vi "post_dust_event_small.vi"(8 "error in (no error)":errorcluster, 11 "Cluster":T1 {"File Location" items=["Currently Writing"=-3, "Labview Files"=-2, "Mars Data Processing Factility"=-1, "Local Cache "=0, "Old Storage"=1, "Storage"=2]; "Estimate Source" items=["Any Source."=-2, "No Shot"=-1, "Basic Labview Estimate"=0, "IDL Estimate From Andrew"=1, "IDL Estimate From Tobin"=2, "Old Metadata"=3]}) -> (0 "error out":errorcluster, 1 "Experiment Settings":i32, 2 "Dust Event ID":i32, 3 "Test Server":bool)   [LabVIEW 2013]
uses:
  Post_Dust_Event_small.ctl
  Private/Estimate_source.ctl
  Private/File_location.ctl
  <vilib>/addons/database/Auxilliary.llb/DB Tools Cursor Type.ctl
  <vilib>/addons/database/Connection.llb/Conn Execute.vi
  <vilib>/addons/database/Recordset.llb/Rec Fetch Recordset Data (R).vi
  <vilib>/addons/database/Recordset.llb/Rec Destroy - Connection.vi
  <vilib>/addons/database/_DB Variant To Data/Database Variant To Data.xnode
  <vilib>/addons/database/NI_Database_API.lvlib
panel:
  # "Dust Event Small"
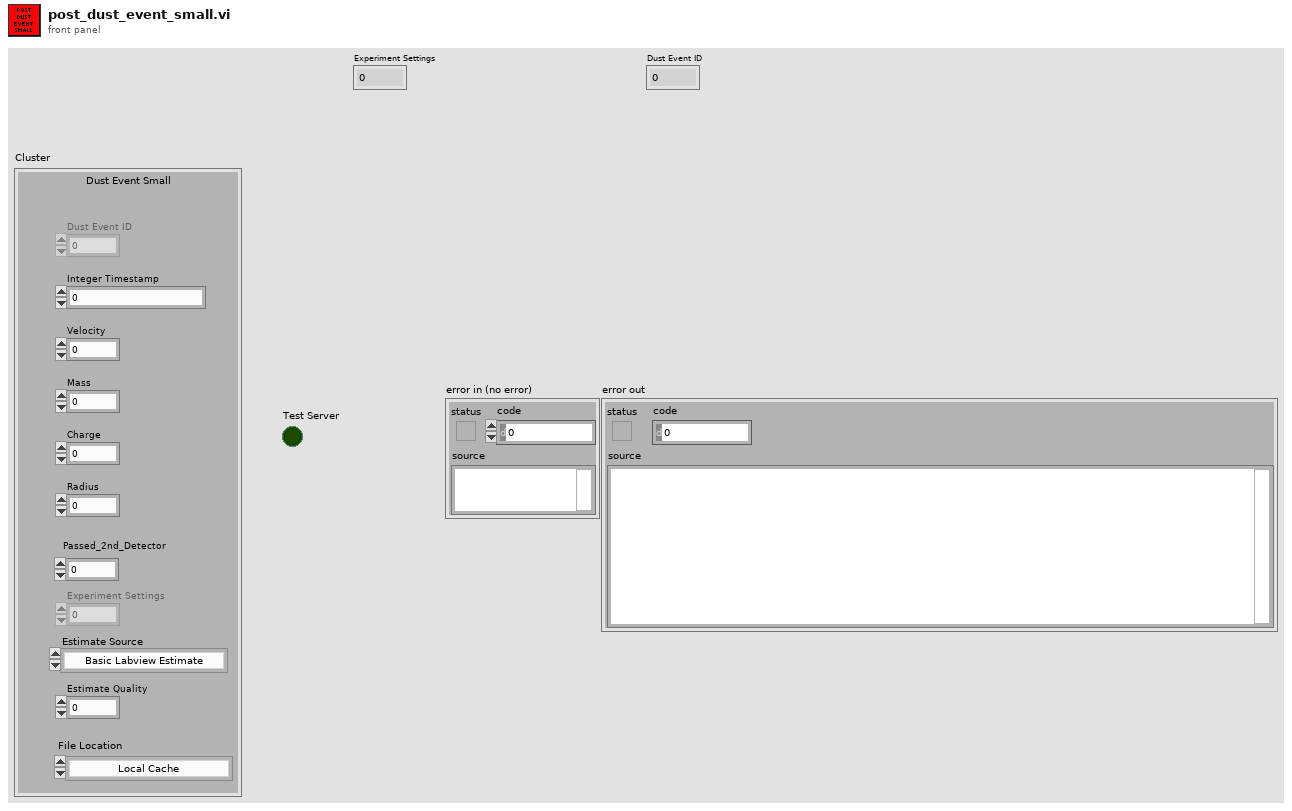
[diagram p1: front panel]
types:
  T1 = typedef "Post_Dust_Event_small.ctl" = cluster{"Dust Event ID":i64, "Integer Timestamp":i64, "Velocity":sgl, "Mass":sgl, "Charge":sgl, "Radius":sgl, "Passed_2nd_Detector":i8, "Experiment Settings":dbl, "Estimate Source":T2, "Estimate Quality":sgl, "File Location":T3, "id_dust_info":dbl}
  T2 = typedef "Estimate_source.ctl" = i8
  T3 = typedef "File_location.ctl" = i8
  T4 = typedef "NI_Database_API.lvlib/DB Tools Cursor Type.ctl" = enum16{"forward-only", "keyset", "dynamic", "static"}
  T5 = typedef "NI_Database_API.lvlib/Conn ObjectReference.ctl" = refnum<k1>
  T6 = typedef "NI_Database_API.lvlib/Rec ObjectReference.ctl" = refnum<k1>
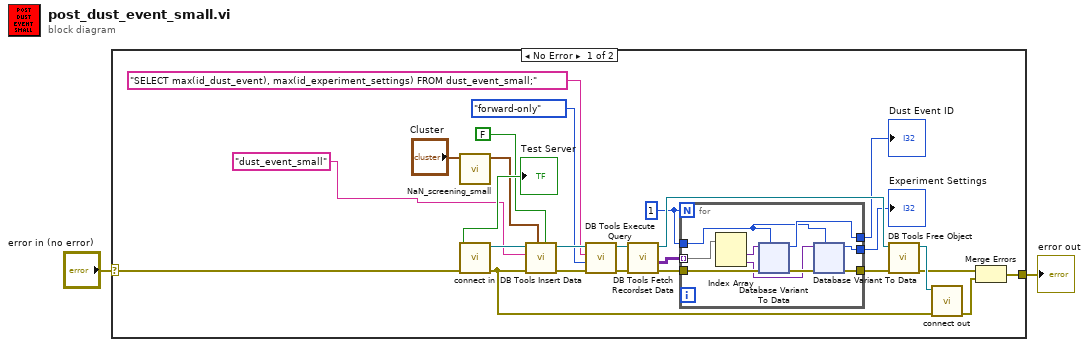
[diagram p0: block diagram]
diagram:
  n1 = case shown="No Error" "error in (no error)" {
    selector: "error in (no error)" -> [w24 w101]
    tunnel: [w21 w101] -> w1
    frame No Error {
      w11 = 1
      n2 = call "NaN_screening_small.vi"("Input"="Cluster") -> ("Output"=w6:T1)  [unwired: 10 in]
      n3 = call "connect in.vi"("error in (no error)"=w24) -> ("error out"=w23:errorcluster, "Database Connection"=w27:T5, "Test Server"=→"Test Server":bool)  [unwired: 6 in]
      n4 = call <vilib>:"DB Tools Insert Data.vi"("create table? (F)"=FALSE, "data"=w6, "error in (no error)"=w23, "table"="dust_event_small", "connection reference"=w27) -> ("error out"=w5:errorcluster, "connection reference out"=w18:T5)  [unwired: 5 in]
      n5 = call-poly <vilib>:"DB Tools Execute Query.vi"("error in (no error)"=w5, "cursor type"=DB_Tools_Cursor_Type."forward-only", "SQL query"="SELECT max(id_dust_event), max(id_experiment_settings) FROM dust_event_small;", "connection reference"=w18) -> ("error out"=w19:errorcluster, "recordset reference"=w20:T6)  [unwired: 4 in]
      n6 = call-poly <vilib>:"DB Tools Fetch Recordset Data.vi"("error in (no error)"=w19, "recordset reference"=w20) -> ("error out"=w9:errorcluster, "recordset data"=w12:variant[][], "recordset reference out"=w17:T6)  [unwired: 3 in]
      n7 = for {
        N: w11 -> [_]
        tunnel: w12 -> [w36] mode=indexing
        tunnel: w11 -> [w30]
        tunnel: [w34] -> w10
        tunnel: [w28] -> w8
        tunnel: w9 -> [w33]
        tunnel: [w29] -> w4
        n8 = Index Array(array=w36) -> (element #1=w35:variant, element #2=w31:variant)  [unwired: 2 in]
        n9 = xnode "Database Variant To Data"("database variant"=w35, "error in"=w33, "type"=w30) -> ("data"=w34:i32, "error out"=w32:errorcluster)
        n10 = xnode "Database Variant To Data"("database variant"=w31, "error in"=w32, "type"=w30) -> ("data"=w29:i32, "error out"=w28:errorcluster)
      }
      "Dust Event ID" <- w10
      "Experiment Settings" <- w4
      n11 = call-poly <vilib>:"DB Tools Free Object.vi"("error in (no error)"=w8, "recordset reference"=w17) -> ("error out"=w15:errorcluster, "connection reference"=w16:T5)  [unwired: 8 in]
      n12 = call "connect out.vi"("error in (no error)"=w23, "connection reference"=w16) -> ("error out"=w22:errorcluster)  [unwired: 9 in]
      n13 = Merge Errors(w15, w22) -> (w21:errorcluster)
    }
    frame Error {
    }
  }
  "error out" <- w1
